vi "From 2D Bool Tree Data.vi"(11 "Tree Data":refnum<class "Tree Data.lvclass">) -> (2 "2D Bool":bool[][](array[boolean]))   [LabVIEW 2020, in "NI_VIAnCFGDataStructure.lvlib" / "2D Bool.lvclass"]
doc: "Extract a 2D Bool value from Tree Data type."
uses:
  <vilib>/addons/analyzer/VIAnCFGDataStructure/Data Types/2D Bool/2D Bool.lvclass
  <vilib>/addons/analyzer/VIAnCFGDataStructure/Tree Data/Tree Data.lvclass
  <vilib>/addons/analyzer/VIAnCFGDataStructure/Data Types/2D Bool/2D Bool.lvclass/2D Bool.ctl
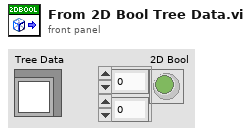
[diagram p1: front panel]
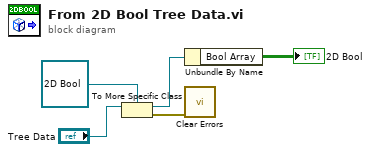
[diagram p0: block diagram]
diagram:
  n1 = To More Specific Class(target class=refnum<class "2D Bool.lvclass"> refnum ("Tree API.lvlib:2D Bool.lvclass"), reference="Tree Data") -> (specific class reference=w3:refnum<class "2D Bool.lvclass">, error out=w2:errorcluster)  [unwired: 1 in]
  n2 = Unbundle By Name(w3) -> ("Bool Array"=→"2D Bool":bool[][])
  n3 = call <vilib>:"Clear Errors.vi"("error in (no error)"=w2) -> ()  [unwired: 5 in, 2 out]
